vi "PathPlanner_Cmd_AutoInitFromAutoFile.vi"(11 "FileName":string="auto.auto") -> (0 "error out":errorcluster, 2 "version":string, 3 "PathPlanner_Cmd_AutoConfig":T1 {"Paths"."IdealStartingState"."Rotation"."SIN" format="%13.4f"; "Paths"."IdealStartingState"."Rotation"."COS" format="%13.4f"; "Paths"."IdealStartingState"."Rotation"."VALUE" format="%13.4f"; "Paths"."PointTowardsZones"."TargetPosition"."Y" format="%14.3f"; "Paths"."PointTowardsZones"."TargetPosition"."X" format="%14.3f"; "Paths"."PointTowardsZones"."RotationOffset"."SIN" format="%13.4f"; "Paths"."PointTowardsZones"."RotationOffset"."COS" format="%13.4f"; "Paths"."PointTowardsZones"."RotationOffset"."VALUE" format="%13.4f"; "Paths"."Waypoints"."nextControl"."Y" format="%14.3f"; "Paths"."Waypoints"."nextControl"."X" format="%14.3f"; "Paths"."Waypoints"."anchor"."Y" format="%14.3f"; "Paths"."Waypoints"."anchor"."X" format="%14.3f"; "Paths"."Waypoints"."prevControl"."Y" format="%14.3f"; "Paths"."Waypoints"."prevControl"."X" format="%14.3f"; "Paths"."AllPoints"."RotationTarget"."rotation"."SIN" format="%13.4f"; "Paths"."AllPoints"."RotationTarget"."rotation"."COS" format="%13.4f"; "Paths"."AllPoints"."RotationTarget"."rotation"."VALUE" format="%13.4f"; "Paths"."AllPoints"."Position"."Y" format="%14.3f"; "Paths"."AllPoints"."Position"."X" format="%14.3f"; "Paths"."GoalEndState"."Rotation"."SIN" format="%13.4f"; "Paths"."GoalEndState"."Rotation"."COS" format="%13.4f"; "Paths"."GoalEndState"."Rotation"."VALUE" format="%13.4f"; "Paths"."RotationTargets"."rotation"."SIN" format="%13.4f"; "Paths"."RotationTargets"."rotation"."COS" format="%13.4f"; "Paths"."RotationTargets"."rotation"."VALUE" format="%13.4f"}, 4 "Full Filename":string)   [LabVIEW 2019, in "PathPlanner24.lvlib"]
doc: "Load an auto from a path file in storage. The path normally has a .AUTO extension. If the file name does not have an extention, the .AUTO is added to the file name. Internally this file is formatted as JSON.\n\nInputs: \n - filename - string - The name of the auto to load\n\nOutputs:\n - PathPlanner_Cmd_AutoConfig - cluster - Configuration created from the contents of the auto file.\n - version - string - Version string from file contents.\n - Error out - cluster - Error cluster\n - Full Filename - string - fully qualified file name.\n\nNotes on file naming:\n - The file name must include the extention. \".auto\" or have no extension. If the filename has no extension, .AUTO is added to the file name.\n - The file name can be a simple file or an absolute path. If a simple file name is used the default path on the RoboRIO is: \"home:\\lvuser\\natinst\\LabVIEW Data\". On a Windows PC the default path is the LabVIEW default directory. Normally this is: “%HOMEDRIVE%%HOMEPATH%\\Documents\\LabView Data\".\n - Filenames on the RoboRIO, which runs Linux, are case sensitive.\n\nNotes:\n--------\nAuto files current processing the following items.\n - Wait\n - Named\n - Path\n - Sequential. Sequential autos may contain, Wait, Named, Path. Other types of commands are ignored.\n - other types of commands are ignored.\n\nThe following table lists the actions performed for different types of commands:\n - Unknown - nothing - not supported.\n - Wait - waits the given amount of time. Drive motor demand is set to zero during this time.\n - Named - Issue boolean command with TRUE value using the \"name\" as the command name.\n - Path - follow the path.\n - Sequential - This is processed as an array of commands given one at a time. Only the above command types are followed."
uses:
  PathPlanner24.lvlib
  TypeDef/PathPlannerCmdPathPlannerAutoConfig.ctl
  TypeDef/PathPlannerCommandUtil.ctl
  ENum/PathPlanner_CommandUtilType_ENUM.ctl
  TypeDef/PathPlannerPath.ctl
  TypeDef/PathPlannerRotationTarget.ctl
  <vilib>/Rock Robotics/WPI/ThirdParty/JAS_Junk/TrajLib/TypeDef/ROTATION2D.ctl
  TypeDef/PathPlannerConstraintsZone.ctl
  TypeDef/PathPlannerPathConstraints.ctl
  TypeDef/PathPlannerEventMarker.ctl
  TypeDef/PathPlannerGoalEndState.ctl
  TypeDef/PathPlannerPathPoint.ctl
  <vilib>/Rock Robotics/WPI/ThirdParty/JAS_Junk/TrajLib/TypeDef/TRANSLATION2D.ctl
  TypeDef/PathPlannerWaypoint.ctl
  TypeDef/PathPlannerPointTowardsZone.ctl
  TypeDef/PathPlannerIdealStartingState.ctl
  PathPlanner_CommandUtil_TypeFromString.vi
  PathPlanner_Cmd_AutoPathsFromCommand.vi
  PathPlanner_Cmd_AutoInitFromJsonData.vi
  PathPlanner_Path_FromPathFile.vi
  <vilib>/Rock Robotics/WPI/ThirdParty/JAS_Junk/TrajLib/Trajectory_Library.lvlib
panel:
  in  "error in (no error)":errorcluster
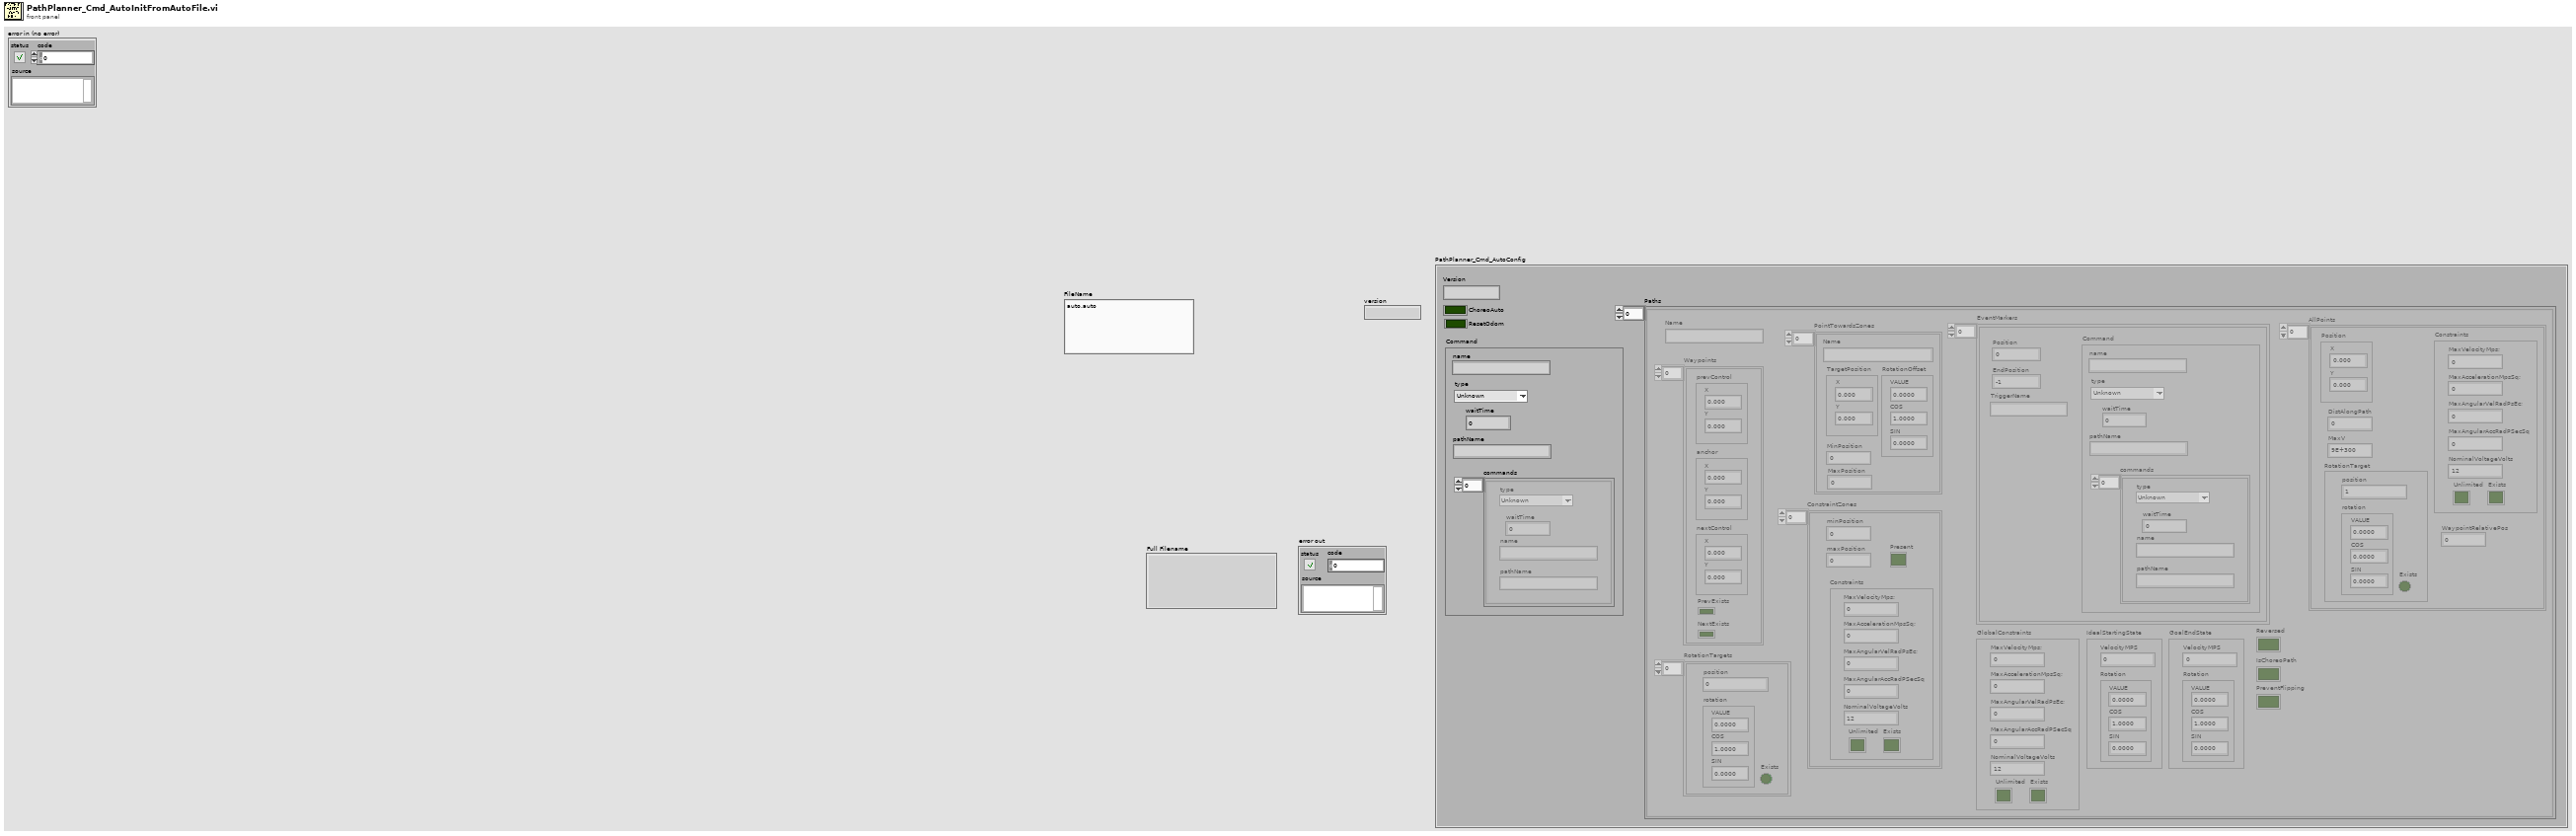
[diagram p1: front panel]
types:
  T1 = typedef "PathPlanner24.lvlib/PathPlannerCmdPathPlannerAutoConfig.ctl" = cluster{"Command":T2, "ChoreoAuto":bool, "Version":string, "ResetOdom":bool, "Paths":T4[]}
  T2 = typedef "PathPlanner24.lvlib/PathPlannerCommandUtil.ctl" = cluster{"waitTime":dbl, "name":string, "pathName":string, "commands":cluster{"type":T3, "waitTime":dbl, "name":string, "pathName":string}[], "type":T3}
  T3 = typedef "PathPlanner24.lvlib/PathPlanner_CommandUtilType_ENUM.ctl" = enum16{"Unknown", "Wait", "Named", "Path", "Sequential", "Parallel", "Race", "Deadline"}
  T4 = typedef "PathPlanner24.lvlib/PathPlannerPath.ctl" = cluster{"Reversed":bool, "RotationTargets":T5[], "ConstraintZones":T7[], "EventMarkers":T9[], "GlobalConstraints":T8, "GoalEndState":T10, "AllPoints":T11[], "Name":string, "Waypoints":T13[], "PointTowardsZones":T14[], "IdealStartingState":T15, "IsChoreoPath":bool, "PreventFlipping":bool}
  T5 = typedef "PathPlanner24.lvlib/PathPlannerRotationTarget.ctl" = cluster{"position":dbl, "rotation":T6, "Exists":bool}
  T6 = typedef "Trajectory_Library.lvlib/ROTATION2D.ctl" = cluster{"VALUE":dbl, "COS":dbl, "SIN":dbl}
  T7 = typedef "PathPlanner24.lvlib/PathPlannerConstraintsZone.ctl" = cluster{"minPosition":dbl, "maxPosition":dbl, "Constraints":T8, "Present":bool}
  T8 = typedef "PathPlanner24.lvlib/PathPlannerPathConstraints.ctl" = cluster{"MaxVelocityMps;":dbl, "MaxAccelerationMpsSq;":dbl, "MaxAngularVelRadPsEc;":dbl, "MaxAngularAccRadPSecSq":dbl, "Exists":bool, "Unlimited":bool, "NominalVoltageVolts":dbl}
  T9 = typedef "PathPlanner24.lvlib/PathPlannerEventMarker.ctl" = cluster{"Position":dbl, "Command":T2, "TriggerName":string, "EndPosition":dbl}
  T10 = typedef "PathPlanner24.lvlib/PathPlannerGoalEndState.ctl" = cluster{"VelocityMPS":dbl, "Rotation":T6}
  T11 = typedef "PathPlanner24.lvlib/PathPlannerPathPoint.ctl" = cluster{"Position":T12, "DistAlongPath":dbl, "MaxV":dbl, "Constraints":T8, "RotationTarget":T5, "WaypointRelativePos":dbl}
  T12 = typedef "Trajectory_Library.lvlib/TRANSLATION2D.ctl" = cluster{"X":dbl, "Y":dbl}
  T13 = typedef "PathPlanner24.lvlib/PathPlannerWaypoint.ctl" = cluster{"prevControl":T12, "anchor":T12, "nextControl":T12, "PrevExists":bool, "NextExists":bool}
  T14 = typedef "PathPlanner24.lvlib/PathPlannerPointTowardsZone.ctl" = cluster{"RotationOffset":T6, "Name":string, "TargetPosition":T12, "MinPosition":dbl, "MaxPosition":dbl}
  T15 = typedef "PathPlanner24.lvlib/PathPlannerIdealStartingState.ctl" = cluster{"VelocityMPS":dbl, "Rotation":T6}
  T16 = enum16{"open", "replace", "create", "open or create", "replace or create", "replace or create with confirmation"}
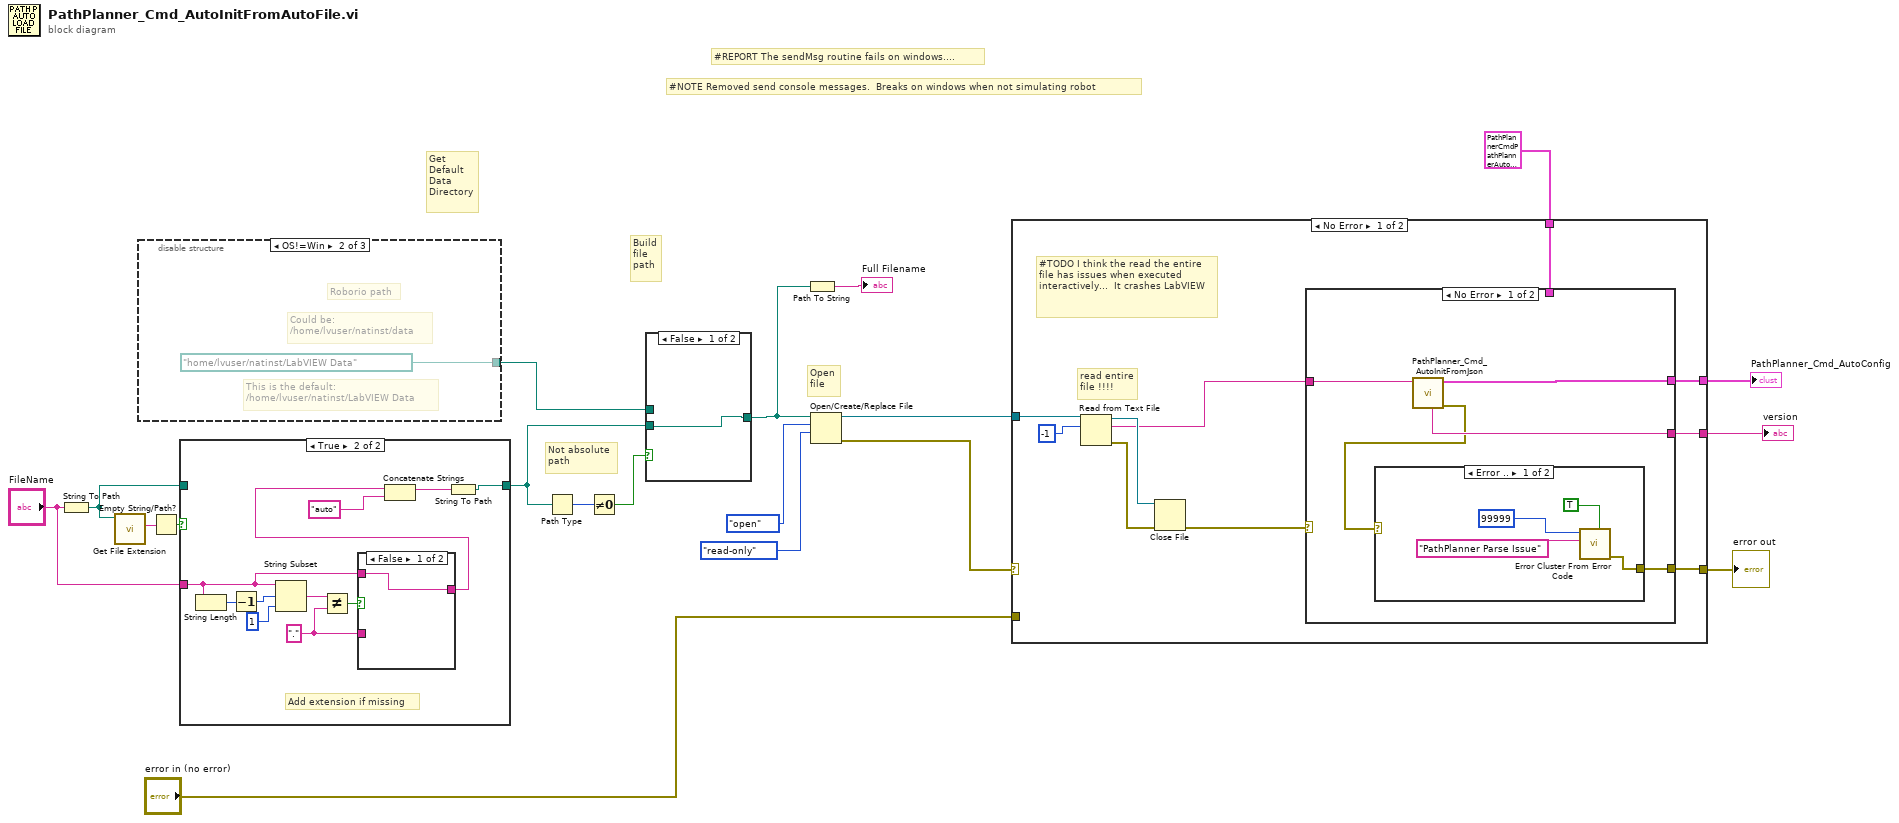
[diagram p0: block diagram]
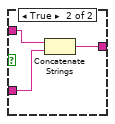
[diagram p3: hidden frame]
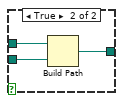
[diagram p4: hidden frame]
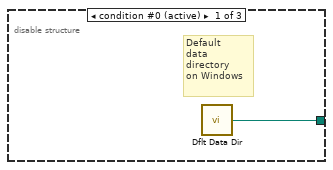
[diagram p5: hidden frame]
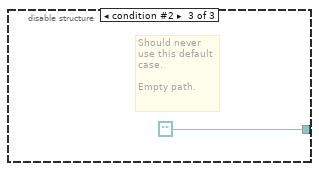
[diagram p6: hidden frame]
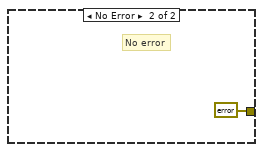
[diagram p7: hidden frame]
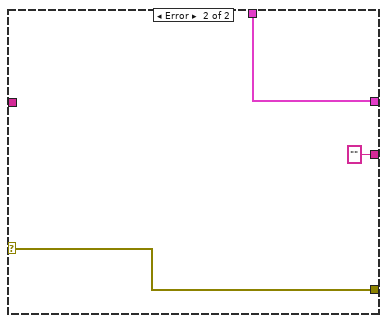
[diagram p8: hidden frame]
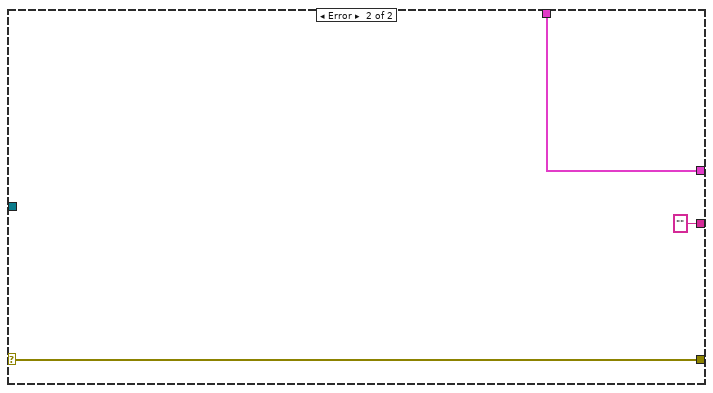
[diagram p9: hidden frame]
diagram:
  # "Not absolute\npath"
  # "#NOTE Removed send console messages.  Breaks on windows when not simulating robot"
  # "#REPORT The sendMsg routine fails on windows...."
  # "Get\nDefault\nData\nDirectory"
  # "Open\nfile"
  # "Build\nfile\npath"
  n1 = String To Path(string="FileName") -> (path=w6:path)
  n2 = call <vilib>:"Get File Extension.vi"("file"=w6) -> ("lowercase file extension"=w4:string)  [unwired: 6 in, 4 out]
  n3 = disable-structure shown="OS!=Win" {
    disable-tunnel: [w20 path "/home/lvuser/natinst/LabVIEW Data" path ""] -> w16
    frame condition #0 (active) {
      # "Default\ndata\ndirectory\non Windows"
      n4 = call <vilib>:"Dflt Data Dir.vi"() -> ("App:Default Data Directory"=w20:path)
    }
    frame condition #1 {
      # "This is the default:\n/home/lvuser/natinst/LabVIEW Data"
      # "Could be:\n/home/lvuser/natinst/data"
      # "Roborio path"
    }
    frame condition #2 {
      # "Should never\nuse this default\ncase.\n\nEmpty path."
    }
  }
  n5 = Empty String/Path?(string/path=w4) -> (empty?=w7:bool)
  n6 = case shown="True" w7 {
    tunnel: w6 -> [w23 _]
    tunnel: [w23 w25] -> w5
    tunnel: "FileName" -> [_ w29]
    frame False {
    }
    frame True {
      w28 = "."
      # "Add extension if missing"
      n7 = String Length(string=w29) -> (length=w34:i32)
      n8 = Decrement(x=w34) -> (x-1=w33:i32)
      n9 = String Subset(string=w29, offset (0)=w33, length (rest)=1 ("length (rest)")) -> (substring=w31:string)
      n10 = Not Equal?(x=w31, y=w28) -> (x != y?=w30:bool)
      n11 = case shown="False" w30 {
        tunnel: w29 -> [w35 w38]
        tunnel: w28 -> [_ w37]
        tunnel: [w35 w36] -> w27
        frame False {
        }
        frame True {
          n12 = Concatenate Strings(w38, w37) -> (w36:string)
        }
      }
      n13 = Concatenate Strings(w27, "auto" ("string")) -> (w24:string)
      n14 = String To Path(string=w24) -> (path=w25:path)
    }
  }
  n15 = Path Type(1:w5) -> (0:w15:i16)
  n16 = Not Equal To 0?(x=w15) -> (x != 0?=w14:bool)
  n17 = case shown="False" w14 {
    tunnel: [w39 w42] -> w11
    tunnel: w16 -> [_ w41]
    tunnel: w5 -> [w39 w40]
    frame False {
    }
    frame True {
      n18 = Build Path(base path=w41, name or relative path=w40) -> (appended path=w42:path)
    }
  }
  n19 = Path To String(path=w11) -> (string=→"Full Filename":string)
  n20 = Open/Create/Replace File(file path (use dialog)=w11, operation (0:open)=T16."open", access (0:read/write)=enum16{"read/write", "read-only", "write-only"}."read-only") -> (refnum out=w12:refnum<file>, error out=w17:errorcluster)  [unwired: 3 in, 1 out]
  n21 = case shown="No Error" w17 {
    selector: w17 -> [_ w68]
    tunnel: w12 -> [w51 _]
    tunnel: [w46 w68] -> w9
    tunnel: "error in (no error)" -> [_ _]
    tunnel: [w45 w66] -> w2
    tunnel: [w44 "" ("version")] -> w8
    tunnel: T1 {"Command"={"waitTime"=0.0, "name"="", "pathName"="", "commands"=[], "type"=enum."Unknown"}, "ChoreoAuto"=FALSE, "Version"="", "ResetOdom"=FALSE, "Paths"=[]} ("PathPlanner_Cmd_AutoConfig") -> [w43 w66]
    frame No Error {
      # "#TODO I think the read the entire\nfile has issues when executed\ninteractively...  It crashes LabVIEW"
      # "read entire\nfile !!!!"
      n22 = Read from Text File(file (use dialog)=w51, count=-1) -> (refnum out=w50:refnum<file>, text=w49:string, error out=w48:errorcluster)  [unwired: 2 in, 1 out]
      n23 = Close File(refnum=w50, error in=w48) -> (error out=w47:errorcluster)  [unwired: 1 out]
      n24 = case shown="No Error" w47 {
        selector: w47 -> [_ w65]
        tunnel: w49 -> [w56 _]
        tunnel: [w57 w65] -> w46
        tunnel: [w55 w63] -> w45
        tunnel: [w54 "" ("version")] -> w44
        tunnel: w43 -> [_ w63]
        frame No Error {
          n25 = call "PathPlanner_Cmd_AutoInitFromJson.vi"("JSON_String"=w56) -> ("error out"=w53:errorcluster, "PathPlanner_Cmd_AutoConfig"=w55:T1, "version"=w54:string)  [unwired: 8 in]
          n26 = case shown="Error .." w53 {
            tunnel: [w58 errorcluster {"status"=FALSE, "code"=0, "source"=""} ("error out")] -> w57
            frame Error {
              n27 = call <vilib>:"Error Cluster From Error Code.vi"("is warning? (False)"=TRUE, "error message (\"\")"="PathPlanner Parse Issue" ("error message (\"\")"), "error code (0)"=99999) -> ("error out"=w58:errorcluster)  [unwired: 6 in]
            }
            frame No Error {
              # "No error"
            }
          }
        }
        frame Error {
        }
      }
    }
    frame Error {
    }
  }
  "error out" <- w9
  "version" <- w8
  "PathPlanner_Cmd_AutoConfig" <- w2
